vi "Mem_U8ArrayToData.vi"(7 "Type":variant, 8 "error in (no error)":errorcluster, 10 "ByteArray":u8[](array[numeric])) -> (0 "error out":errorcluster, 1 "Supported Type?":bool, 2 "data":variant, 4 "ByteArray Left":u8[](array[numeric]))   [LabVIEW 2019, in "Memory Data Access.lvlib"]
uses:
  Memory Data Access.lvlib
  <vilib>/Utility/Data Type/Type Definitions/Data Type.ctl
  <vilib>/Utility/Data Type/NI_Data Type.lvlib
panel:
  out "*(type *) &x":dbl[](array[numeric])
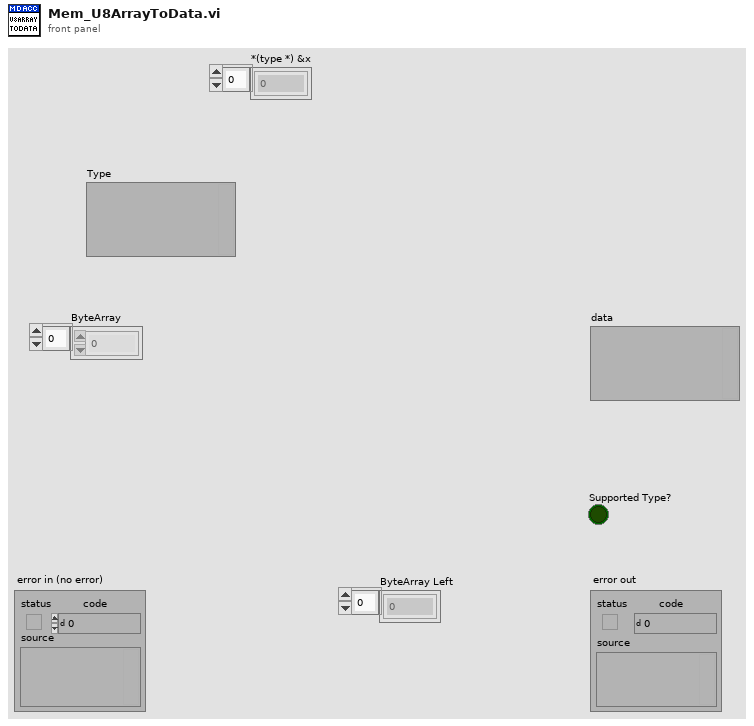
[diagram p1: front panel]
types:
  T1 = typedef "NI_Data Type.lvlib/Data Type.ctl" = enum8{"Invalid Type", "Void", "I8", "I16", "I32", "I64", "U8", "U16", "U32", "U64", "Single Float", "Double Float", "Extended Float", "Single Complex", "Double Complex", "Extended Complex", "Enum U8", "Enum U16", "Enum U32", "Enum U64", "Single Float With Unit", "Double Float With Unit", "Extended Float With Unit", "Single Complex with Unit", "Double Complex with Unit", "Extended Complex with Unit", "Boolean", "String", "Path", "Picture", "Tag", "Array", "Cluster", "Variant", "LV Variant", "Waveform", "Timestamp", "Digital Waveform", "Digital Data", "ExpressData", "Refnum", "External Data", "VI", "Poly VI", "LabVIEW Class Instance", "Fixed Point", "Set Collection", "Map Collection"}
  T2 = typedef "Type Descriptor Enumeration__ogtk.ctl" = enum8{"<Null>", "I8", "I16", "I32", "I64", "U8", "U16", "U32", "U64", "SGL", "DBL", "EXT", "CSG", "CDB", "CXT", "0x0F", "0x10", "0x11", "0x12", "0x13", "0x14", "Enum U8", "Enum U16", "Enum U32", "Enum U64", "SGL PQ", "DBL PQ", "EXT PQ", "CSG PQ", "CDB PQ", "CXT PQ", "0x1F", "0x20", "Boolean", "0x22", "0x23", "0x24", "0x25", "0x26", "0x27", "0x28", "0x29", "0x2A", "0x2B", "0x2C", "0x2D", "0x2E", "0x2F", "String", "0x31", "Path", "Pict", "0x34", "0x35", "0x36", "DAQ", "0x38", "0x39", "0x3A", "0x3B", "0x3C", "0x3D", "0x3E", "0x3F", "Array", "0x41", "0x42", "0x43", "0x44", "0x45", "0x46", "0x47", "0x48", "0x49", "0x4A", "0x4B", "0x4C", "0x4D", "0x4E", "0x4F", "Cluster", "0x51", "0x52", "Variant", "Waveform", "0x55", "0x56", "0x57", "0x58", "0x59", "0x5A", "0x5B", "0x5C", "0x5D", "0x5E", "0x5F", "0x60", "0x61", "0x62", "0x63", "0x64", "0x65", "0x66", "0x67", "0x68", "0x69", "0x6A", "0x6B", "0x6C", "0x6D", "0x6E", "0x6F", "Refnum"}
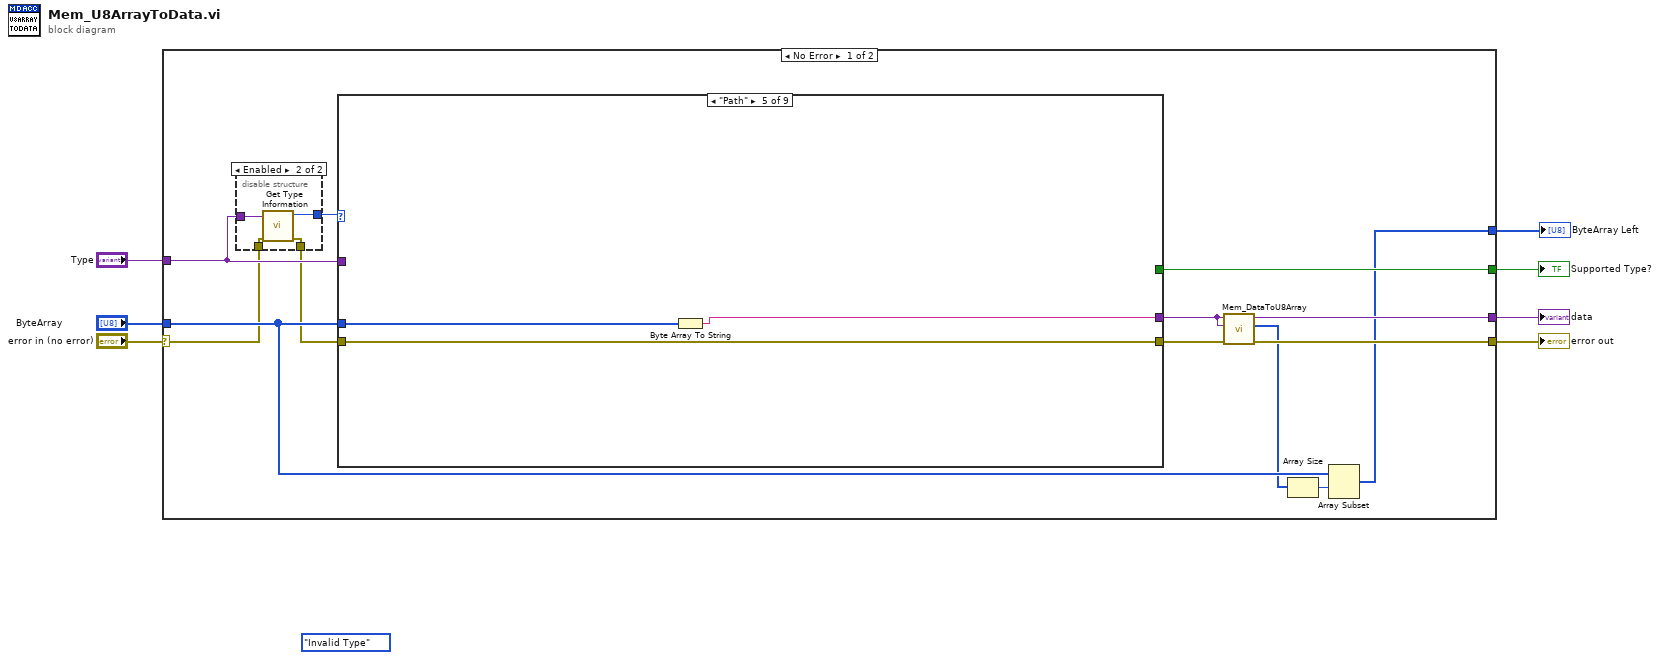
[diagram p0: block diagram]
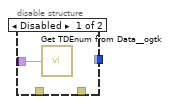
[diagram p2: hidden frame]
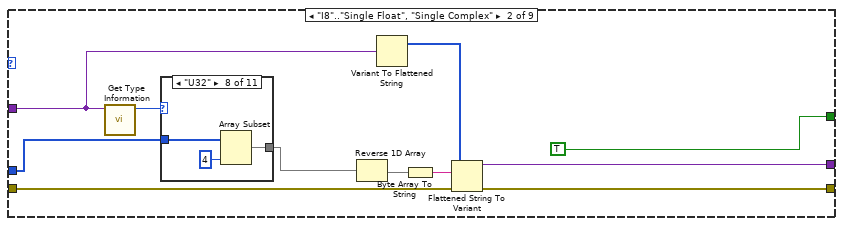
[diagram p4: hidden frame]
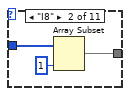
[diagram p6: hidden frame]
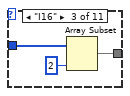
[diagram p7: hidden frame]
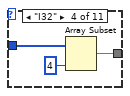
[diagram p8: hidden frame]
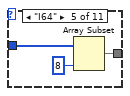
[diagram p9: hidden frame]
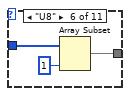
[diagram p10: hidden frame]
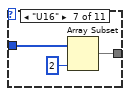
[diagram p11: hidden frame]
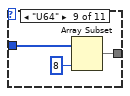
[diagram p12: hidden frame]
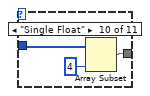
[diagram p13: hidden frame]
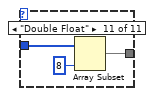
[diagram p14: hidden frame]
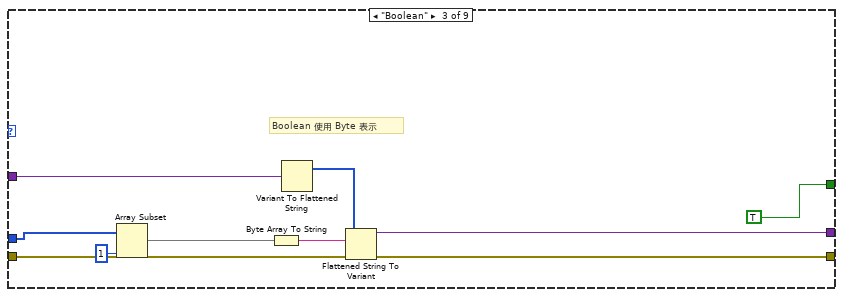
[diagram p15: hidden frame]
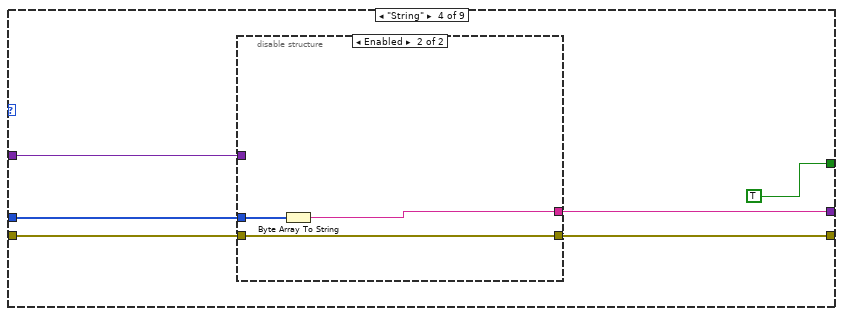
[diagram p16: hidden frame]
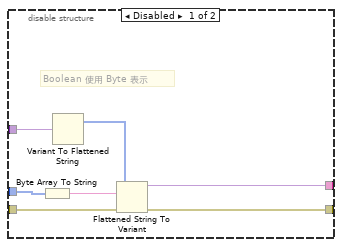
[diagram p17: hidden frame]
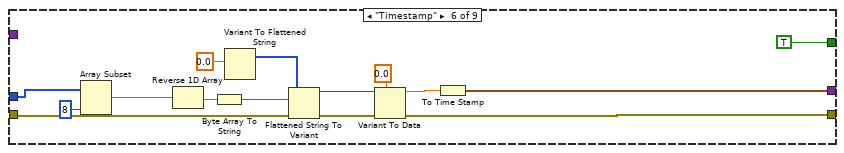
[diagram p18: hidden frame]
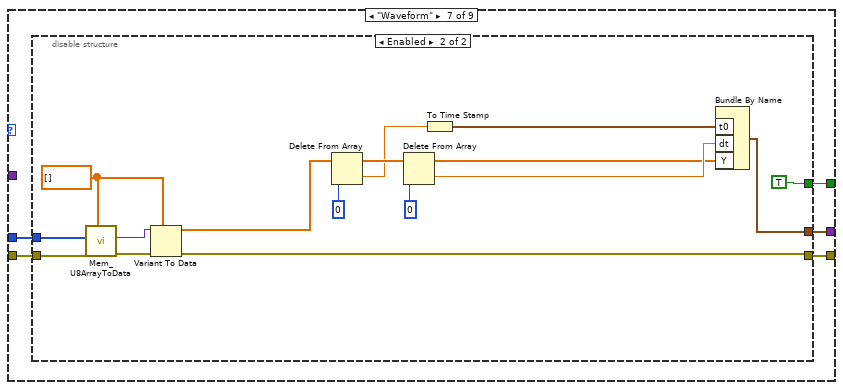
[diagram p19: hidden frame]
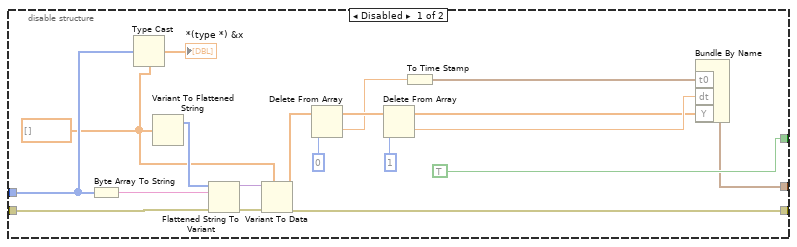
[diagram p20: hidden frame]
diagram:
  (unwired) Data_Type."Invalid Type" ("type")
  n1 = case shown="No Error" "error in (no error)" {
    selector: "error in (no error)" -> [w9 w493]
    tunnel: "ByteArray" -> [w14 _]
    tunnel: [w16 w493] -> w5
    tunnel: "Type" -> [w19 w492]
    tunnel: [w15 w492] -> w3
    tunnel: [w18 _] -> w2
    tunnel: [w13 _] -> w1
    frame No Error {
      n2 = disable-structure shown="Enabled" {
        disable-tunnel: w19 -> [w20 w25]
        disable-tunnel: [_ w24] -> w10
        disable-tunnel: w9 -> [_ w23]
        disable-tunnel: [_ w22] -> w8
        frame Disabled {
          n3 = call <userlib>:"Get TDEnum from Data__ogtk.vi"("Data"=w20) -> ("Type Descriptor Enumeration"=w21:T2)  [unwired: 4 in]
        }
        frame Enabled {
          n4 = call <vilib>:"Get Type Information.vi"("error in (no error)"=w23, "variant"=w25) -> ("error out"=w22:errorcluster, "type"=w24:T1)  [unwired: 5 in, 3 out]
        }
      }
      n5 = case shown="\"Path\"" w10 {
        tunnel: w8 -> [w27 w31 w76 w82 w97 w110 w117 w163 w416]
        tunnel: [w27 w36 w75 w81 w97 w103 w116 w160 w418] -> w17
        tunnel: w19 -> [w26 w28 w78 w84 _ _ _ w164 w421]
        tunnel: [_ TRUE TRUE TRUE _ TRUE w118 w161 w424] -> w18
        tunnel: w14 -> [_ w30 w71 w83 w98 w100 w114 w158 w422]
        tunnel: [w26 w35 w74 w80 w96 w104 w115 w159 w413] -> w15
        frame "Invalid Type", Default {
        }
        frame "I8".."Single Float", "Single Complex" {
          n6 = call <vilib>:"Get Type Information.vi"("variant"=w28) -> ("type"=w32:T1)  [unwired: 6 in, 4 out]
          n7 = case shown="\"U32\"" w32 {
            tunnel: w30 -> [w39 w42 w44 w47 w50 w53 w56 w59 w62 w65 w68]
            tunnel: [w39 w40 w43 w46 w49 w52 w55 w58 w61 w64 w67] -> w29
            frame "Invalid Type", Default {
            }
            frame "I8" {
              n8 = Array Subset(array=w42, length=1) -> (w40:u8[])  [unwired: 1 in]
            }
            frame "I16" {
              n9 = Array Subset(array=w44, length=2) -> (w43:u8[])  [unwired: 1 in]
            }
            frame "I32" {
              n10 = Array Subset(array=w47, length=4) -> (w46:u8[])  [unwired: 1 in]
            }
            frame "I64" {
              n11 = Array Subset(array=w50, length=8) -> (w49:u8[])  [unwired: 1 in]
            }
            frame "U8" {
              n12 = Array Subset(array=w53, length=1) -> (w52:u8[])  [unwired: 1 in]
            }
            frame "U16" {
              n13 = Array Subset(array=w56, length=2) -> (w55:u8[])  [unwired: 1 in]
            }
            frame "U32" {
              n14 = Array Subset(array=w59, length=4) -> (w58:u8[])  [unwired: 1 in]
            }
            frame "U64" {
              n15 = Array Subset(array=w62, length=8) -> (w61:u8[])  [unwired: 1 in]
            }
            frame "Single Float" {
              n16 = Array Subset(array=w65, length=4) -> (w64:u8[])  [unwired: 1 in]
            }
            frame "Double Float" {
              n17 = Array Subset(array=w68, length=8) -> (w67:u8[])  [unwired: 1 in]
            }
          }
          n18 = Reverse 1D Array(array=w29) -> (reversed array=w33:u8[])
          n19 = Variant To Flattened String(Variant=w28) -> (1:w37:i16[])  [unwired: 1 out]
          n20 = Byte Array To String(unsigned byte array=w33) -> (string=w34:string)
          n21 = Flattened String To Variant(4:w31, 6:w34, 7:w37) -> (0:w36:errorcluster, 3:w35:variant)
        }
        frame "Boolean" {
          # "Boolean 使用 Byte 表示"
          n22 = Array Subset(array=w71, length=1) -> (w70:u8[])  [unwired: 1 in]
          n23 = Byte Array To String(unsigned byte array=w70) -> (string=w73:string)
          n24 = Variant To Flattened String(Variant=w78) -> (1:w77:i16[])  [unwired: 1 out]
          n25 = Flattened String To Variant(4:w76, 6:w73, 7:w77) -> (0:w75:errorcluster, 3:w74:variant)
        }
        frame "String" {
          n26 = disable-structure shown="Enabled" {
            disable-tunnel: w84 -> [w92 _]
            disable-tunnel: w83 -> [w90 w95]
            disable-tunnel: w82 -> [w89 w94]
            disable-tunnel: [w88 w94] -> w81
            disable-tunnel: [w87 w93] -> w80
            frame Disabled {
              # "Boolean 使用 Byte 表示"
              n27 = Byte Array To String(unsigned byte array=w90) -> (string=w86:string)
              n28 = Variant To Flattened String(Variant=w92) -> (1:w91:i16[])  [unwired: 1 out]
              n29 = Flattened String To Variant(4:w89, 6:w86, 7:w91) -> (0:w88:errorcluster, 3:w87:variant)
            }
            frame Enabled {
              n30 = Byte Array To String(unsigned byte array=w95) -> (string=w93:string)
            }
          }
        }
        frame "Path" {
          n31 = Byte Array To String(unsigned byte array=w98) -> (string=w96:string)
        }
        frame "Timestamp" {
          n32 = Array Subset(array=w100, length=8) -> (w99:u8[])  [unwired: 1 in]
          n33 = Reverse 1D Array(array=w99) -> (reversed array=w111:u8[])
          n34 = Byte Array To String(unsigned byte array=w111) -> (string=w112:string)
          n35 = Variant To Flattened String(Variant=0.0) -> (1:w113:i16[])  [unwired: 1 out]
          n36 = Flattened String To Variant(4:w110, 6:w112, 7:w113) -> (0:w107:errorcluster, 3:w108:variant)
          n37 = Variant To Data(error in=w107, type=0.0, Variant=w108) -> (data=w105:dbl, error out=w103:errorcluster)
          n38 = To Time Stamp(1:w105) -> (0:w104:timestamp)
        }
        frame "Waveform" {
          n39 = disable-structure shown="Enabled" {
            disable-tunnel: [TRUE TRUE] -> w118
            disable-tunnel: w117 -> [w135 w145]
            disable-tunnel: [w133 w139] -> w116
            disable-tunnel: [w123 w141] -> w115
            disable-tunnel: w114 -> [w121 w146]
            frame Disabled {
              w120 = dbl[] [] ("array")
              n40 = Byte Array To String(unsigned byte array=w121) -> (string=w122:string)
              n41 = Type Cast(type=w120, x=w121) -> (*(type *) &x=→"*(type *) &x":dbl[])
              n42 = Variant To Flattened String(Variant=w120) -> (1:w136:i16[])  [unwired: 1 out]
              n43 = Flattened String To Variant(4:w135, 6:w122, 7:w136) -> (0:w134:errorcluster, 3:w132:variant)
              n44 = Variant To Data(error in=w134, type=w120, Variant=w132) -> (data=w131:dbl[], error out=w133:errorcluster)
              n45 = Delete From Array(array=w131, index=0) -> (deleted portion=w127:dbl, array with subset deleted=w130:dbl[])  [unwired: 1 in]
              n46 = Delete From Array(array=w130, index=1) -> (deleted portion=w125:dbl, array with subset deleted=w124:dbl[])  [unwired: 1 in]
              n47 = To Time Stamp(1:w127) -> (0:w126:timestamp)
              n48 = Bundle By Name("t0"=w126, "dt"=w125, "Y"=w124) -> (w123:waveform(dbl))  [unwired: 1 in]
            }
            frame Enabled {
              w138 = dbl[] [] ("array")
              n49 = call "Mem_U8ArrayToData.vi"("Type"=w138, "error in (no error)"=w145, "ByteArray"=w146) -> ("error out"=w143:errorcluster, "data"=w144:variant)  [unwired: 5 in, 2 out]
              n50 = Variant To Data(error in=w143, type=w138, Variant=w144) -> (data=w142:dbl[], error out=w139:errorcluster)
              n51 = Delete From Array(array=w142, index=0) -> (deleted portion=w150:dbl, array with subset deleted=w153:dbl[])  [unwired: 1 in]
              n52 = Delete From Array(array=w153, index=0) -> (deleted portion=w148:dbl, array with subset deleted=w147:dbl[])  [unwired: 1 in]
              n53 = To Time Stamp(1:w150) -> (0:w149:timestamp)
              n54 = Bundle By Name("t0"=w149, "dt"=w148, "Y"=w147) -> (w141:waveform(dbl))  [unwired: 1 in]
            }
          }
        }
        frame "Array" {
          n55 = call <vilib>:"Get Array Information.vi"("error in (no error)"=w163, "variant"=w164) -> ("error out"=w162:errorcluster, "array element data type"=w157:variant)  [unwired: 6 in, 2 out]
          n56 = call "Mem_DataToU8Array.vi"("error in (no error)"=w162, "Payload"=w157) -> ("error out"=w155:errorcluster, "Supported Type?"=w161:bool)  [unwired: 7 in, 1 out]
          n57 = call <vilib>:"Get Type Information.vi"("error in (no error)"=w155, "variant"=w157) -> ("error out"=w156:errorcluster, "type"=w154:T1)  [unwired: 5 in, 3 out]
          n58 = case shown="\"String\"" w154 {
            tunnel: w164 -> [_ _ _ _ _ _ _ _ _ _ _ w385]
            tunnel: w156 -> [w169 w185 w202 w222 w241 w261 w283 w302 w322 w343 w363 w384]
            tunnel: [w166 w183 w202 w222 w241 w261 w283 w302 w322 w343 w363 w383] -> w160
            tunnel: [w165 w184 w201 w221 w242 w262 w281 w301 w321 w341 w361 w382] -> w159
            tunnel: w158 -> [w174 w186 w203 w223 w243 w263 w282 w303 w323 w342 w362 w381]
            frame "Waveform" {
              w172 = u32 0 ("offset (0)")
              n59 = call "Mem_U8ArrayToData.vi"("Type"=w172, "error in (no error)"=w169, "ByteArray"=w174) -> ("error out"=w171:errorcluster, "data"=w173:variant, "ByteArray Left"=w168:u8[])  [unwired: 5 in, 1 out]
              n60 = Variant To Data(error in=w171, type=w172, Variant=w173) -> (data=w170:u32, error out=w167:errorcluster)
              n61 = for {
                N: w170 -> [_]
                shift-right: [w177] -> w166
                shift-left: w167 -> [w181]
                tunnel: [w178] -> w165 mode=indexing
                shift-right: [w175] -> _
                shift-left: w168 -> [w182]
                w179 = waveform(dbl) {"t0"=timestamp(0 s since 1904-01-01), "dt"=1.0, "Y"=[]} ("Waveform")
                n62 = call "Mem_U8ArrayToData.vi"("Type"=w179, "error in (no error)"=w181, "ByteArray"=w182) -> ("error out"=w176:errorcluster, "data"=w180:variant, "ByteArray Left"=w175:u8[])  [unwired: 5 in, 1 out]
                n63 = Variant To Data(error in=w176, type=w179, Variant=w180) -> (data=w178:waveform(dbl), error out=w177:errorcluster)
              }
            }
            frame "String" {
              w191 = u32 0 ("offset (0)")
              n64 = call "Mem_U8ArrayToData.vi"("Type"=w191, "error in (no error)"=w185, "ByteArray"=w186) -> ("error out"=w190:errorcluster, "data"=w192:variant, "ByteArray Left"=w188:u8[])  [unwired: 5 in, 1 out]
              n65 = Variant To Data(error in=w190, type=w191, Variant=w192) -> (data=w189:u32, error out=w187:errorcluster)
              n66 = for {
                N: w189 -> [_]
                shift-right: [w196] -> w183
                shift-left: w187 -> [w199]
                tunnel: [w197] -> w184 mode=indexing
                shift-right: [w194] -> _
                shift-left: w188 -> [w200]
                w193 = ""
                n67 = call "Mem_U8ArrayToData.vi"("Type"=w193, "error in (no error)"=w199, "ByteArray"=w200) -> ("error out"=w195:errorcluster, "data"=w198:variant, "ByteArray Left"=w194:u8[])  [unwired: 5 in, 1 out]
                n68 = Variant To Data(error in=w195, type=w193, Variant=w198) -> (data=w197:string, error out=w196:errorcluster)
              }
            }
            frame "I8" {
              n69 = Array Subset(array=w203, index=0, length=4) -> (w206:u8[])
              n70 = Reverse 1D Array(array=w206) -> (reversed array=w210:u8[])
              n71 = Type Cast(type=u32 0, x=w210) -> (*(type *) &x=w208:u32)
              n72 = for {
                N: w208 -> [_]
                tunnel: w203 -> [w220]
                tunnel: [w211] -> w209 mode=indexing
                i -> [w219]
                w218 = 1 ("length")
                n73 = Multiply(x=w218, y=w219) -> (x*y=w217:i32)
                n74 = Add(x=4 ("length"), y=w217) -> (x+y=w215:i32)
                n75 = Array Subset(array=w220, index=w215, length=w218) -> (w214:u8[])
                n76 = Reverse 1D Array(array=w214) -> (reversed array=w213:u8[])
                n77 = Type Cast(type=i8 0, x=w213) -> (*(type *) &x=w211:i8)
              }
              n78 = To Variant(anything=w209) -> (Variant=w201:variant)
            }
            frame "I16" {
              n79 = Array Subset(array=w223, index=0, length=4) -> (w226:u8[])
              n80 = Reverse 1D Array(array=w226) -> (reversed array=w230:u8[])
              n81 = Type Cast(type=u32 0, x=w230) -> (*(type *) &x=w228:u32)
              n82 = for {
                N: w228 -> [_]
                tunnel: w223 -> [w240]
                tunnel: [w231] -> w229 mode=indexing
                i -> [w239]
                w238 = 2 ("length")
                n83 = Multiply(x=w238, y=w239) -> (x*y=w237:i32)
                n84 = Add(x=4 ("length"), y=w237) -> (x+y=w235:i32)
                n85 = Array Subset(array=w240, index=w235, length=w238) -> (w234:u8[])
                n86 = Reverse 1D Array(array=w234) -> (reversed array=w233:u8[])
                n87 = Type Cast(type=i16 0, x=w233) -> (*(type *) &x=w231:i16)
              }
              n88 = To Variant(anything=w229) -> (Variant=w221:variant)
            }
            frame "I32" {
              n89 = Array Subset(array=w243, index=0, length=4) -> (w246:u8[])
              n90 = Reverse 1D Array(array=w246) -> (reversed array=w250:u8[])
              n91 = Type Cast(type=u32 0, x=w250) -> (*(type *) &x=w248:u32)
              n92 = for {
                N: w248 -> [_]
                tunnel: w243 -> [w260]
                tunnel: [w251] -> w249 mode=indexing
                i -> [w259]
                w258 = 4 ("length")
                n93 = Multiply(x=w258, y=w259) -> (x*y=w257:i32)
                n94 = Add(x=4 ("length"), y=w257) -> (x+y=w255:i32)
                n95 = Array Subset(array=w260, index=w255, length=w258) -> (w254:u8[])
                n96 = Reverse 1D Array(array=w254) -> (reversed array=w253:u8[])
                n97 = Type Cast(type=0, x=w253) -> (*(type *) &x=w251:i32)
              }
              n98 = To Variant(anything=w249) -> (Variant=w242:variant)
            }
            frame "I64" {
              n99 = Array Subset(array=w263, index=0, length=4) -> (w266:u8[])
              n100 = Reverse 1D Array(array=w266) -> (reversed array=w270:u8[])
              n101 = Type Cast(type=u32 0, x=w270) -> (*(type *) &x=w268:u32)
              n102 = for {
                N: w268 -> [_]
                tunnel: w263 -> [w280]
                tunnel: [w271] -> w269 mode=indexing
                i -> [w279]
                w278 = 8 ("length")
                n103 = Multiply(x=w278, y=w279) -> (x*y=w277:i32)
                n104 = Add(x=4 ("length"), y=w277) -> (x+y=w275:i32)
                n105 = Array Subset(array=w280, index=w275, length=w278) -> (w274:u8[])
                n106 = Reverse 1D Array(array=w274) -> (reversed array=w273:u8[])
                n107 = Type Cast(type=i64 0, x=w273) -> (*(type *) &x=w271:i64)
              }
              n108 = To Variant(anything=w269) -> (Variant=w262:variant)
            }
            frame "U8" {
              n109 = Array Subset(array=w282, index=0, length=4) -> (w286:u8[])
              n110 = Reverse 1D Array(array=w286) -> (reversed array=w290:u8[])
              n111 = Type Cast(type=u32 0, x=w290) -> (*(type *) &x=w288:u32)
              n112 = for {
                N: w288 -> [_]
                tunnel: w282 -> [w300]
                tunnel: [w291] -> w289 mode=indexing
                i -> [w299]
                w298 = 1 ("length")
                n113 = Multiply(x=w298, y=w299) -> (x*y=w297:i32)
                n114 = Add(x=4 ("length"), y=w297) -> (x+y=w295:i32)
                n115 = Array Subset(array=w300, index=w295, length=w298) -> (w294:u8[])
                n116 = Reverse 1D Array(array=w294) -> (reversed array=w293:u8[])
                n117 = Type Cast(type=u8 0, x=w293) -> (*(type *) &x=w291:u8)
              }
              n118 = To Variant(anything=w289) -> (Variant=w281:variant)
            }
            frame "U16" {
              n119 = Array Subset(array=w303, index=0, length=4) -> (w306:u8[])
              n120 = Reverse 1D Array(array=w306) -> (reversed array=w310:u8[])
              n121 = Type Cast(type=u32 0, x=w310) -> (*(type *) &x=w308:u32)
              n122 = for {
                N: w308 -> [_]
                tunnel: w303 -> [w320]
                tunnel: [w311] -> w309 mode=indexing
                i -> [w319]
                w318 = 2 ("length")
                n123 = Multiply(x=w318, y=w319) -> (x*y=w317:i32)
                n124 = Add(x=4 ("length"), y=w317) -> (x+y=w315:i32)
                n125 = Array Subset(array=w320, index=w315, length=w318) -> (w314:u8[])
                n126 = Reverse 1D Array(array=w314) -> (reversed array=w313:u8[])
                n127 = Type Cast(type=u16 0, x=w313) -> (*(type *) &x=w311:u16)
              }
              n128 = To Variant(anything=w309) -> (Variant=w301:variant)
            }
            frame "U32" {
              n129 = Array Subset(array=w323, index=0, length=4) -> (w326:u8[])
              n130 = Reverse 1D Array(array=w326) -> (reversed array=w330:u8[])
              n131 = Type Cast(type=u32 0, x=w330) -> (*(type *) &x=w328:u32)
              n132 = for {
                N: w328 -> [_]
                tunnel: w323 -> [w340]
                tunnel: [w331] -> w329 mode=indexing
                i -> [w339]
                w338 = 4 ("length")
                n133 = Multiply(x=w338, y=w339) -> (x*y=w337:i32)
                n134 = Add(x=4 ("length"), y=w337) -> (x+y=w335:i32)
                n135 = Array Subset(array=w340, index=w335, length=w338) -> (w334:u8[])
                n136 = Reverse 1D Array(array=w334) -> (reversed array=w333:u8[])
                n137 = Type Cast(type=u32 0, x=w333) -> (*(type *) &x=w331:u32)
              }
              n138 = To Variant(anything=w329) -> (Variant=w321:variant)
            }
            frame "U64" {
              n139 = Array Subset(array=w342, index=0, length=4) -> (w346:u8[])
              n140 = Reverse 1D Array(array=w346) -> (reversed array=w350:u8[])
              n141 = Type Cast(type=u32 0, x=w350) -> (*(type *) &x=w348:u32)
              n142 = for {
                N: w348 -> [_]
                tunnel: w342 -> [w360]
                tunnel: [w351] -> w349 mode=indexing
                i -> [w359]
                w358 = 8 ("length")
                n143 = Multiply(x=w358, y=w359) -> (x*y=w357:i32)
                n144 = Add(x=4 ("length"), y=w357) -> (x+y=w355:i32)
                n145 = Array Subset(array=w360, index=w355, length=w358) -> (w354:u8[])
                n146 = Reverse 1D Array(array=w354) -> (reversed array=w353:u8[])
                n147 = Type Cast(type=u64 0, x=w353) -> (*(type *) &x=w351:u64)
              }
              n148 = To Variant(anything=w349) -> (Variant=w341:variant)
            }
            frame "Single Float" {
              n149 = Array Subset(array=w362, index=0, length=4) -> (w366:u8[])
              n150 = Reverse 1D Array(array=w366) -> (reversed array=w370:u8[])
              n151 = Type Cast(type=u32 0, x=w370) -> (*(type *) &x=w368:u32)
              n152 = for {
                N: w368 -> [_]
                tunnel: w362 -> [w380]
                tunnel: [w371] -> w369 mode=indexing
                i -> [w379]
                w378 = 4 ("length")
                n153 = Multiply(x=w378, y=w379) -> (x*y=w377:i32)
                n154 = Add(x=4 ("length"), y=w377) -> (x+y=w375:i32)
                n155 = Array Subset(array=w380, index=w375, length=w378) -> (w374:u8[])
                n156 = Reverse 1D Array(array=w374) -> (reversed array=w373:u8[])
                n157 = Type Cast(type=sgl 0.0, x=w373) -> (*(type *) &x=w371:sgl)
              }
              n158 = To Variant(anything=w369) -> (Variant=w361:variant)
            }
            frame "Double Float", Default {
              n159 = disable-structure shown="Enabled" {
                disable-tunnel: w385 -> [w392 _]
                disable-tunnel: w384 -> [w390 w394]
                disable-tunnel: [w389 w394] -> w383
                disable-tunnel: [w388 w396] -> w382
                disable-tunnel: w381 -> [w387 w397]
                frame Disabled {
                  n160 = Byte Array To String(unsigned byte array=w387) -> (string=w386:string)
                  n161 = Variant To Flattened String(Variant=w392) -> (1:w391:i16[])  [unwired: 1 out]
                  n162 = Flattened String To Variant(4:w390, 6:w386, 7:w391) -> (0:w389:errorcluster, 3:w388:variant)
                }
                frame Enabled {
                  n163 = Array Subset(array=w397, index=0, length=4) -> (w400:u8[])
                  n164 = Reverse 1D Array(array=w400) -> (reversed array=w393:u8[])
                  n165 = Type Cast(type=u32 0, x=w393) -> (*(type *) &x=w398:u32)
                  n166 = for {
                    N: w398 -> [_]
                    tunnel: w397 -> [w412]
                    tunnel: [w403] -> w395 mode=indexing
                    i -> [w411]
                    w410 = 8 ("length")
                    n167 = Multiply(x=w410, y=w411) -> (x*y=w409:i32)
                    n168 = Add(x=4 ("length"), y=w409) -> (x+y=w407:i32)
                    n169 = Array Subset(array=w412, index=w407, length=w410) -> (w406:u8[])
                    n170 = Reverse 1D Array(array=w406) -> (reversed array=w405:u8[])
                    n171 = Type Cast(type=0.0, x=w405) -> (*(type *) &x=w403:dbl)
                  }
                  n172 = To Variant(anything=w395) -> (Variant=w396:variant)
                }
              }
            }
          }
        }
        frame "Cluster" {
          n173 = call <userlib>:"Get Data Name__ogtk.vi"("error in (no error)"=w416, "Data"=w421) -> ("error out"=w417:errorcluster, "Data Name"=w415:string, "Data dup"=w414:variant)  [unwired: 7 in]
          n174 = call <userlib>:"Cluster to Array of VData__ogtk.vi"("error in (no error)"=w417, "Cluster"=w414) -> ("error out"=w423:errorcluster, "Array of VData"=w426:variant[])  [unwired: 8 in]
          n175 = for {
            tunnel: w426 -> [w431] mode=indexing
            tunnel: [w435] -> w425 mode=indexing
            shift-right: [w436] -> w419
            shift-left: w423 -> [w427]
            shift-right: [w433] -> _
            shift-left: w422 -> [w429]
            tunnel: [w434] -> w420 mode=indexing
            n176 = disable-structure shown="Enabled" {
              disable-tunnel: [w439 w442] -> w432
              disable-tunnel: w431 -> [w439 w443]
              disable-tunnel: [w438 w440] -> w430
              disable-tunnel: w429 -> [w438 w444]
              disable-tunnel: [w437 w441] -> w428
              disable-tunnel: w427 -> [w437 w441]
              frame Enabled {
              }
              frame Disabled {
                n177 = call <vilib>:"Get Type Information.vi"("variant"=w443) -> ("type"=w445:T1)  [unwired: 6 in, 4 out]
                n178 = case shown="\"Boolean\"" w445 {
                  tunnel: w444 -> [w446 w451 w454 w458 w462 w466 w470 w474 w478 w482 w486 w490]
                  tunnel: w443 -> [w447 w449 w453 w456 w461 w464 w468 w472 w476 w480 w484 w488]
                  tunnel: [w447 w449 w453 w456 w461 w464 w468 w472 w476 w480 w484 w488] -> w442
                  tunnel: [w446 w448 w452 w457 w460 w465 w469 w473 w477 w481 w485 w489] -> w440
                  frame "Invalid Type", Default {
                  }
                  frame "I8" {
                    n179 = Array Subset(array=w451, length=1) -> (w448:u8[])  [unwired: 1 in]
                  }
                  frame "I16" {
                    n180 = Array Subset(array=w454, length=2) -> (w452:u8[])  [unwired: 1 in]
                  }
                  frame "I32" {
                    n181 = Array Subset(array=w458, length=4) -> (w457:u8[])  [unwired: 1 in]
                  }
                  frame "I64" {
                    n182 = Array Subset(array=w462, length=8) -> (w460:u8[])  [unwired: 1 in]
                  }
                  frame "U8" {
                    n183 = Array Subset(array=w466, length=1) -> (w465:u8[])  [unwired: 1 in]
                  }
                  frame "U16" {
                    n184 = Array Subset(array=w470, length=2) -> (w469:u8[])  [unwired: 1 in]
                  }
                  frame "U32" {
                    n185 = Array Subset(array=w474, length=4) -> (w473:u8[])  [unwired: 1 in]
                  }
                  frame "U64" {
                    n186 = Array Subset(array=w478, length=8) -> (w477:u8[])  [unwired: 1 in]
                  }
                  frame "Single Float" {
                    n187 = Array Subset(array=w482, length=4) -> (w481:u8[])  [unwired: 1 in]
                  }
                  frame "Double Float" {
                    n188 = Array Subset(array=w486, length=2) -> (w485:u8[])  [unwired: 1 in]
                  }
                  frame "Boolean" {
                    n189 = Array Subset(array=w490, length=1) -> (w489:u8[])  [unwired: 1 in]
                  }
                }
              }
            }
            n190 = call "Mem_U8ArrayToData.vi"("Type"=w432, "error in (no error)"=w428, "ByteArray"=w430) -> ("error out"=w436:errorcluster, "Supported Type?"=w435:bool, "data"=w434:variant, "ByteArray Left"=w433:u8[])  [unwired: 5 in]
          }
          n191 = call <userlib>:"Array of VData to VCluster__ogtk.vi"("error in (no error)"=w419, "Cluster Name"=w415, "Array"=w420) -> ("error out"=w418:errorcluster, "VCluster"=w413:variant)  [unwired: 7 in]
          n192 = And Array Elements(Boolean array=w425) -> (logical AND=w424:bool)
        }
      }
      n193 = call "Mem_DataToU8Array.vi"("error in (no error)"=w17, "Payload"=w15) -> ("error out"=w16:errorcluster, "ByteArray"=w12:u8[])  [unwired: 7 in, 1 out]
      n194 = Array Size(array=w12) -> (size(s)=w11:i32)
      n195 = Array Subset(array=w14, index=w11) -> (w13:u8[])  [unwired: 1 in]
    }
    frame Error {
    }
  }
  "error out" <- w5
  "data" <- w3
  "Supported Type?" <- w2
  "ByteArray Left" <- w1
